vi "Handle Module Status.vi"(8 "error in (no error)":errorcluster, 10 "Module Status":T1, 11 "Volatus Core in":refnum<class "Volatus Core.lvclass">) -> (0 "error out":errorcluster, 3 "Volatus Core out":refnum<class "Volatus Core.lvclass">)   [LabVIEW 2020, in "Volatus.lvlib" / "Volatus Core.lvclass"]
uses:
  Volatus Core.lvclass
  C:/dev/lv20CE/relink/lv-volatus/Volatus/Module/Module.lvclass
  Module/Module Status Update.ctl
  MessageQ/MessageQ.lvclass
  Module/State.ctl
  Volatus Core.lvclass/Volatus Core.ctl
  Module/Module.lvclass
  <vilib>/Utility/miscctls.llb/LVMapReplaceAction.ctl
  C:/dev/lv20CE/relink/lv-volatus/Volatus/Volatus Core/Volatus Core.lvclass
  Volatus.lvlib
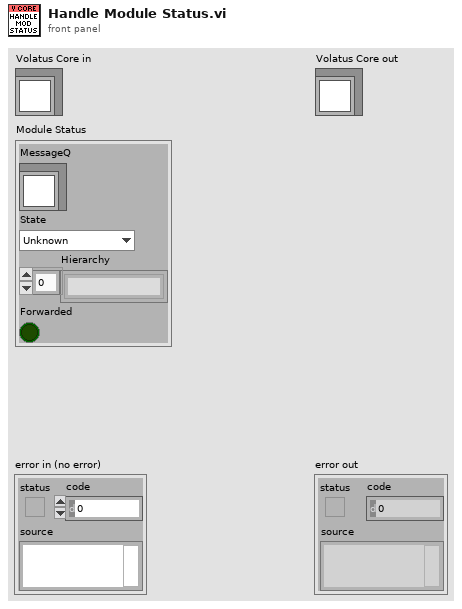
[diagram p1: front panel]
types:
  T1 = typedef "Volatus.lvlib/Module Status Update.ctl" = cluster{"MessageQ":refnum<class "MessageQ.lvclass">, "State":T2, "Hierarchy":string[], "Forwarded":bool}
  T2 = typedef "Volatus.lvlib/Module.lvclass/State.ctl" = enum16{"Unknown", "Launched", "Starting", "Running", "Stopping", "Stopped", "Error - Starting", "Error - Run", "Error - Stopping"}
  T3 = typedef "LVMapReplaceAction.ctl" = enum32{"Modify Entry only if found", "Add or Modify Entry", "Delete Entry"}
  T4 = typedef "Volatus.lvlib/Module Status.ctl" = cluster{"Hierarchy":string[], "State":T2, "Substatus":map{string, string}}
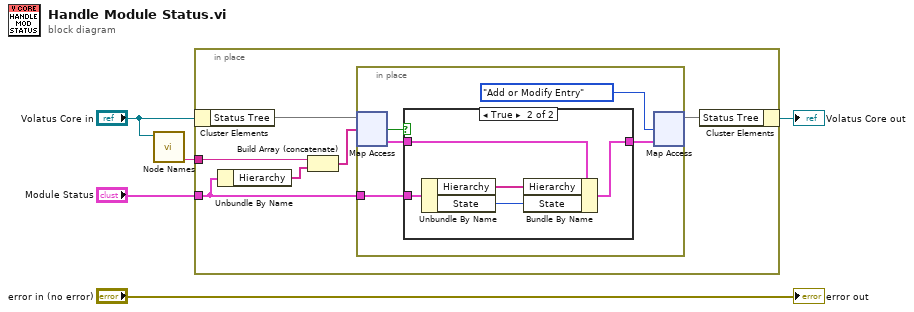
[diagram p0: block diagram]
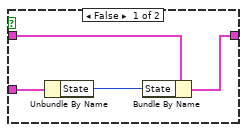
[diagram p2: hidden frame]
diagram:
  n1 = call "Node Names.vi"("Module in"="Volatus Core in") -> ("Node"=w1:string)  [unwired: 6 in, 4 out]
  n2 = in-place {
    in-place-border: "Module Status" -> [w9]
    in-place-border: w1 -> [w10]
    n3 = in-place-cluster #1("Volatus Core in") -> ("Status Tree"=w8:map{string[], T4})
    n4 = Unbundle By Name(w9) -> ("Hierarchy"=w11:string[])
    n5 = Build Array (concatenate)(w10, w11) -> (w7:string[])
    n6 = in-place {
      in-place-border: w9 -> [w14]
      n7 = in-place-map #2(w8, w7) -> (w16:T4, w15:bool)  [unwired: 1 in]
      n8 = case shown="True" w15 {
        tunnel: w16 -> [w20 w25]
        tunnel: w14 -> [w19 w24]
        tunnel: [w17 w21] -> w13
        frame False {
          n9 = Unbundle By Name(w19) -> ("State"=w18:T2)
          n10 = Bundle By Name(cluster=w20, "State"=w18) -> (w17:T4)
        }
        frame True {
          n11 = Unbundle By Name(w24) -> ("Hierarchy"=w23:string[], "State"=w22:T2)
          n12 = Bundle By Name(cluster=w25, "Hierarchy"=w23, "State"=w22) -> (w21:T4)
        }
      }
      n13 = in-place-map #2(w13, LVMapReplaceAction."Add or Modify Entry" ("action")) -> (w6:map{string[], T4})  [unwired: 2 out]
    }
    n14 = in-place-cluster #1("Status Tree"=w6) -> (→"Volatus Core out":refnum<class "Volatus Core.lvclass">)
  }
  "error out" <- "error in (no error)"
